vi "SendToThingspeak.vi"(8 "error in (no error)":errorcluster, 9 "input in":dbl, 10 "Api Key":string, 11 "format string":string) -> (0 "error out":errorcluster)   [LabVIEW 2019]
uses:
  <vilib>/httpClient/LabVIEWHTTPClient.lvlib
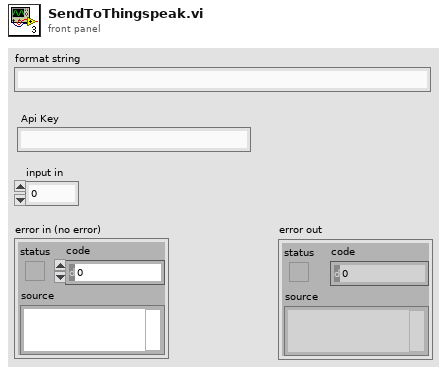
[diagram p1: front panel]
types:
  T1 = typedef "LabVIEWHTTPClient.lvlib/ClientHandle.ctl" = refnum<k1>
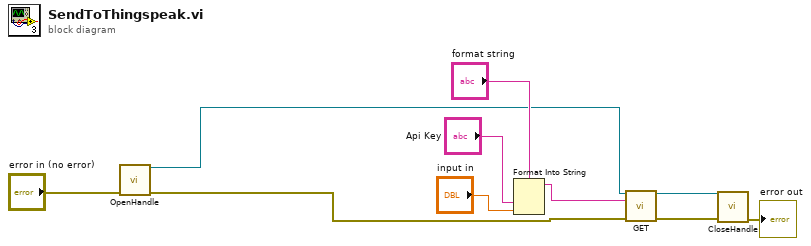
[diagram p0: block diagram]
diagram:
  n1 = call <vilib>:"OpenHandle.vi"("error in (no error)"="error in (no error)") -> ("client handle out"=w8:T1, "error out"=w7:errorcluster)  [unwired: 13 in]
  n2 = Format Into String(format string="format string", "Api Key", "input in") -> (resulting string=w2:string)  [unwired: 2 in, 1 out]
  n3 = call <vilib>:"GET.vi"("client handle"=w8, "url"=w2, "error in (no error)"=w7) -> ("client handle out"=w5:T1, "error out"=w6:errorcluster)  [unwired: 9 in, 2 out]
  n4 = call <vilib>:"CloseHandle.vi"("client handle"=w5, "error in (no error)"=w6) -> ("error out"=→"error out":errorcluster)  [unwired: 13 in]
